vi "MB Registers Write DI.vi"(5 "Data Reference":T1, 8 "error in (no error)":errorcluster, 9 "Bits In":bool[](array[boolean]), 11 "Start Address":u16) -> (0 "error out":errorcluster)   [LabVIEW 2019, in "NI_modbus_upd.lvlib"]
uses:
  Ctl/Data Reference.ctl
  NI_modbus_upd.lvlib
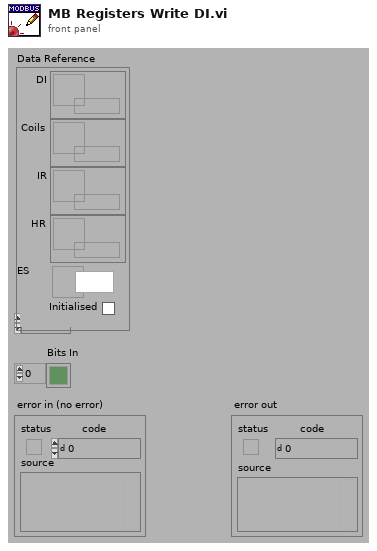
[diagram p1: front panel]
types:
  T1 = typedef "NI_modbus_upd.lvlib/Data Reference.ctl" = cluster{"DI":refnum<data-value>, "Coils":refnum<data-value>, "IR":refnum<data-value>, "HR":refnum<data-value>, "ES":refnum<data-value>, "Initialised":bool}
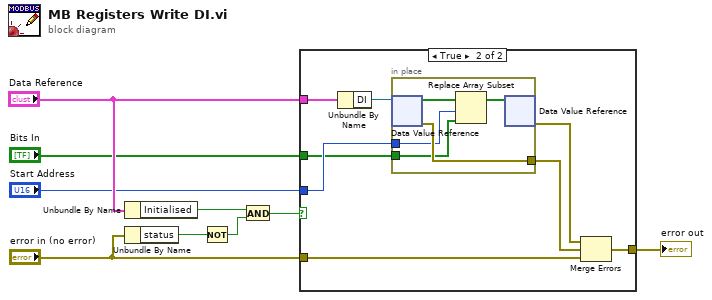
[diagram p0: block diagram]
diagram:
  n1 = Unbundle By Name("Data Reference") -> ("Initialised"=w7:bool)
  n2 = Unbundle By Name("error in (no error)") -> ("status"=w9:bool)
  n3 = Not(x=w9) -> (.not. x?=w8:bool)
  n4 = And(x=w7, y=w8) -> (x .and. y?=w2:bool)
  n5 = case shown="True" w2 {
    tunnel: [w10 w15] -> w3
    tunnel: "Start Address" -> [_ w18]
    tunnel: "Data Reference" -> [_ w17]
    tunnel: "error in (no error)" -> [w10 w16]
    tunnel: "Bits In" -> [_ w14]
    frame False {
    }
    frame True {
      n6 = Unbundle By Name(w17) -> ("DI"=w11:refnum<data-value>)
      n7 = in-place {
        in-place-border: w18 -> [w20]
        in-place-border: [w23] -> w12
        in-place-border: w14 -> [w19]
        n8 = in-place-dvr #1(w11) -> (w22:bool[], w23:errorcluster)
        n9 = Replace Array Subset(array=w22, new element=w19, index=w20) -> (w21:bool[])
        n10 = in-place-dvr #1(w21) -> (w13:errorcluster)  [unwired: 1 out]
      }
      n11 = Merge Errors(w13, w12, w16) -> (w15:errorcluster)
    }
  }
  "error out" <- w3
